vi "Nested Unique.vi"(10 "Nested Alias":string, 11 "Queue Actor in":refnum<class "Queue Actor.lvclass">) -> (2 "Nested Alias Unique?":bool)   [LabVIEW 2021, in "Queue Actor.lvclass"]
uses:
  Queue Actor.lvclass
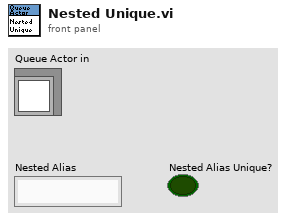
[diagram p1: front panel]
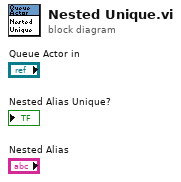
[diagram p0: block diagram]
diagram:
